vi "uClient_GetBroker.vi"(8 "error in (no error)":errorcluster, 11 "uClient in":refnum<class "uClient.lvclass">) -> (0 "error out":errorcluster, 2 "Broker Transport":refnum<class "uTransport_uActor.lvclass">, 3 "uClient out":refnum<class "uClient.lvclass">)   [LabVIEW 2023, in "uLib.lvlib" / "uClient.lvclass"]
uses:
  uClient.lvclass
  uTransport/uTransport_uActor/uTransport_uActor.lvclass
  uClient.lvclass/uClient.ctl
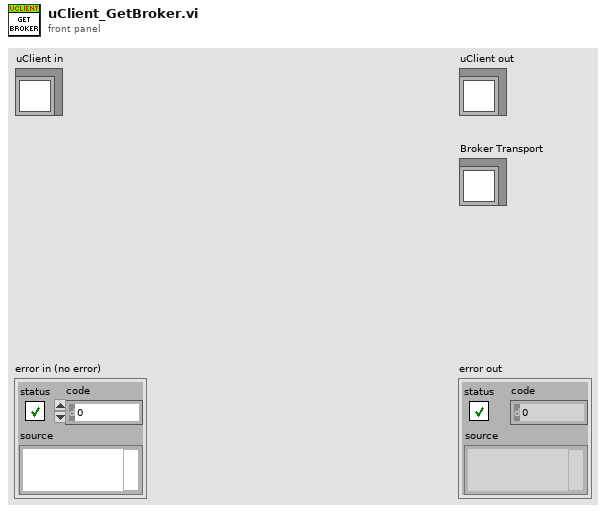
[diagram p1: front panel]
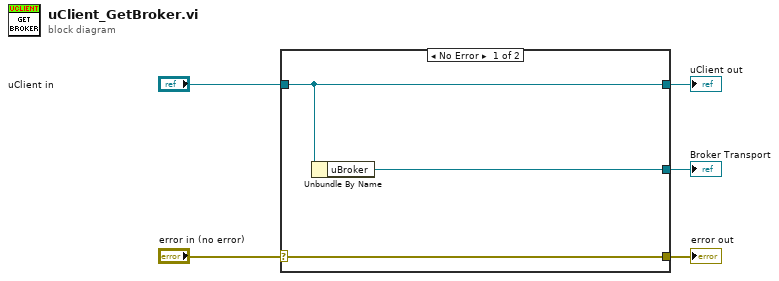
[diagram p0: block diagram]
diagram:
  n1 = case shown="No Error" "error in (no error)" {
    selector: "error in (no error)" -> [w8 w9]
    tunnel: [w8 w9] -> w4
    tunnel: [w7 w10] -> w2
    tunnel: "uClient in" -> [w7 w10]
    tunnel: [w6 _] -> w1
    frame No Error {
      n2 = Unbundle By Name(w7) -> ("uBroker"=w6:refnum<class "uTransport_uActor.lvclass">)
    }
    frame Error {
    }
  }
  "error out" <- w4
  "uClient out" <- w2
  "Broker Transport" <- w1
